vi "Set Modified Flag.vi"(8 "error in (no error)":errorcluster, 11 "Controller in":refnum<class "Controller.lvclass">) -> (0 "error out":errorcluster, 3 "Controller out":refnum<class "Controller.lvclass">)   [LabVIEW 2013, in "SET Project Editor.lvlib" / "Controller.lvclass"]
uses:
  Controller.lvclass
  Controller.lvclass/Controller.ctl
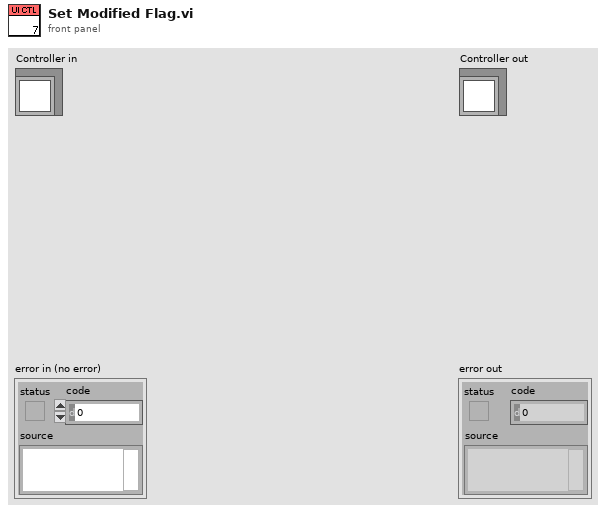
[diagram p1: front panel]
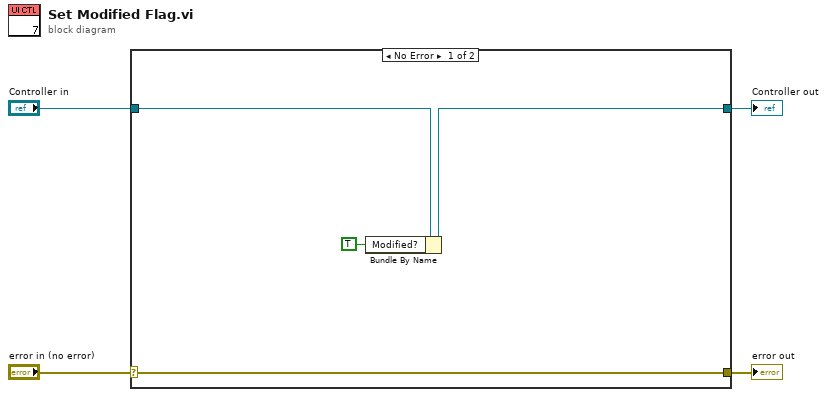
[diagram p0: block diagram]
diagram:
  n1 = case shown="No Error" "error in (no error)" {
    selector: "error in (no error)" -> [w8 w10]
    tunnel: [w8 w10] -> w3
    tunnel: [w6 w9] -> w1
    tunnel: "Controller in" -> [w7 w9]
    frame No Error {
      n2 = Bundle By Name(cluster=w7, "Modified?"=TRUE) -> (w6:refnum<class "Controller.lvclass">)
    }
    frame Error {
    }
  }
  "error out" <- w3
  "Controller out" <- w1
